vi "LaserCTIOTFInterfaceOnOffFGV.vi"(8 "error in":errorcluster, 10 "Set_Get":enum16{"Set", "Get"}(ring), 11 "LaserCtiotfInterfaceOnOffIN":T1) -> (0 "error out":errorcluster, 3 "LaserCtiotfInterfaceOnOffOUT":T1)   [LabVIEW 2010]
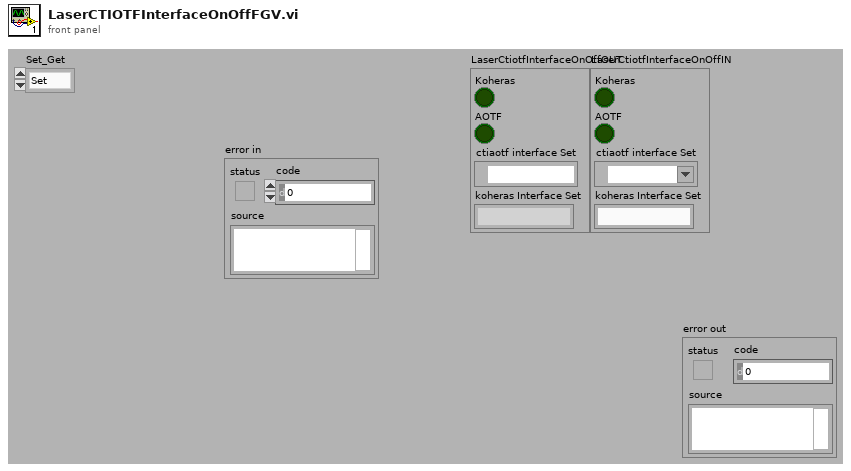
[diagram p1: front panel]
types:
  T1 = cluster{"Koheras":bool, "AOTF":bool, "ctiaotf interface Set":refnum<visa-resource-name>, "koheras Interface Set":string}
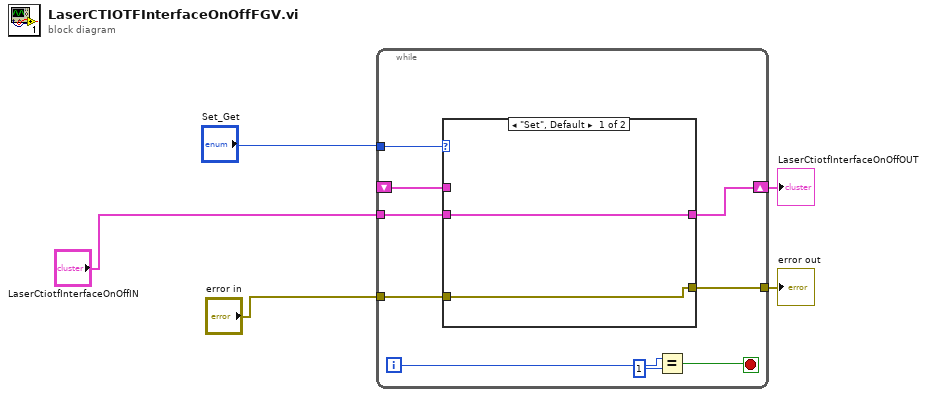
[diagram p0: block diagram]
diagram:
  n1 = while {
    tunnel: "Set_Get" -> [w14]
    tunnel: "LaserCtiotfInterfaceOnOffIN" -> [w13]
    shift-right: [w12] -> w2
    shift-left: _ -> [w11]
    tunnel: "error in" -> [w7]
    tunnel: [w6] -> w3
    i -> [w9]
    stop <- w10 stop-if-true
    n2 = case shown="\"Set\", Default" w14 {
      tunnel: w13 -> [w16 _]
      tunnel: [w16 w18] -> w12
      tunnel: w11 -> [_ w18]
      tunnel: [w15 w17] -> w6
      tunnel: w7 -> [w15 w17]
      frame "Set", Default {
      }
      frame "Get" {
      }
    }
    n3 = Equal?(x=w9, y=1) -> (x = y?=w10:bool)
  }
  "error out" <- w3
  "LaserCtiotfInterfaceOnOffOUT" <- w2
